vi "day1_test1.vi"() -> ()   [LabVIEW 2014]
panel:
  out "출력 변수 2":dbl
  out "출력 변수":dbl
  in  "입력 변수 3":dbl
  in  "입력 변수 2":dbl
  in  "입력 변수":dbl
  out "숫자형 4":dbl format="%#_12g"
  in  "숫자형 3":dbl
  out "Result":dbl
  in  "A6":dbl
  in  "A5":dbl
  in  "A4":dbl
  in  "A3":dbl
  in  "A2":dbl
  in  "A1":dbl
  out "sqrt(x)":dbl
  out "Z":dbl
  in  "Y":dbl
  in  "X":dbl
  out "x != 0?":bool
  out "숫자형 2":dbl format="%#_30g"
  in  "숫자형":dbl
  in  "탭 컨트롤":enum32{"Add/Sub", "Mul/Div"}(tab)
  in  "Input 1":dbl
  in  "Input 2":dbl
  out "Sum":dbl
  out "Difference":dbl
  in  "A":dbl
  in  "B":dbl
  out "ADD":dbl
  out "MUL 2":dbl
  out "Difference":dbl
  out "DIV":dbl format="%#_2f"
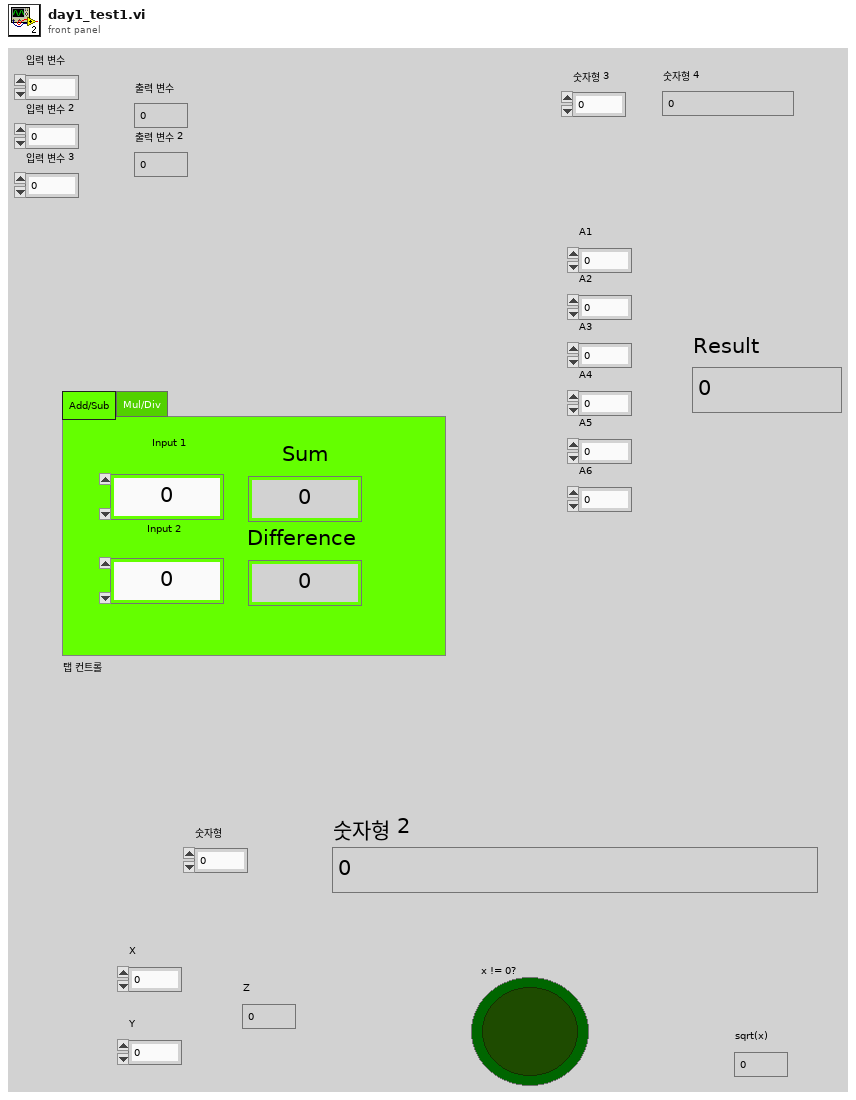
[diagram p1: front panel]
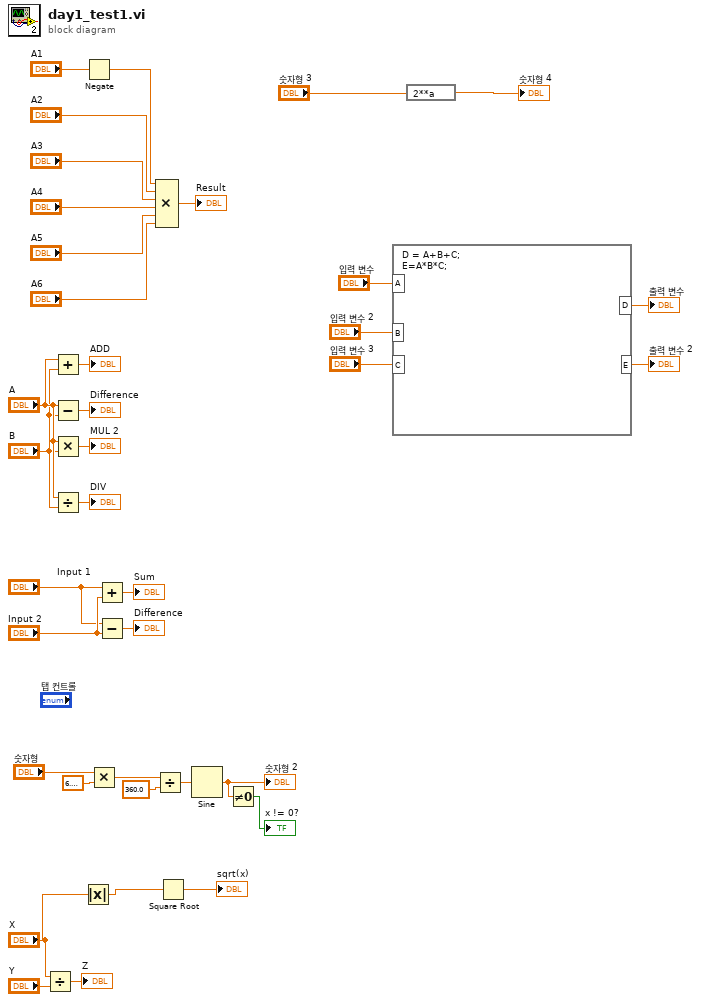
[diagram p0: block diagram]
diagram:
  n1 = Divide(x="X", y="Y") -> (x/y=→"Z":dbl)
  n2 = Add(x="A", y="B") -> (x+y=→"ADD":dbl)
  n3 = Subtract(x="A", y="B") -> (x-y=→"Difference":dbl)
  n4 = Multiply(x="A", y="B") -> (x*y=→"MUL 2":dbl)
  n5 = Divide(x="A", y="B") -> (x/y=→"DIV":dbl)
  n6 = Absolute Value(x="X") -> (abs(x)=w17:dbl)
  n7 = Negate(x="A1") -> (-x=w8:dbl)
  n8 = Multiply(x="숫자형", y=6.283185307179586) -> (x*y=w26:dbl)
  n9 = Add(x="Input 1", y="Input 2") -> (x+y=→"Sum":dbl)
  n10 = Subtract(x="Input 1", y="Input 2") -> (x-y=→"Difference":dbl)
  n11 = Divide(x=w26, y=360.0) -> (x/y=w24:dbl)
  n12 = Compound Arithmetic op=MULTIPLY(w8, "A2", "A3", "A4", "A5", "A6") -> (→"Result":dbl)
  n13 = Square Root(x=w17) -> (sqrt(x)=→"sqrt(x)":dbl)
  n14 = Sine(x=w24) -> (sin(x)=w22:dbl)
  "숫자형 2" <- w22
  n15 = Not Equal To 0?(x=w22) -> (x != 0?=→"x != 0?":bool)
  n16 = formula code="D = A+B+C;\nE=A*B*C;"("A"="입력 변수", "B"="입력 변수 2", "C"="입력 변수 3") -> ("D"=→"출력 변수":dbl, "E"=→"출력 변수 2":dbl)
  n17 = expression code="2**a"("숫자형 3") -> (→"숫자형 4":dbl)
